vi "ResetMedia.vi"(8 "error in (no error)":errorcluster, 11 "UI Refs":T1) -> (0 "error out":errorcluster, 3 "UI Refs":T1)   [LabVIEW 2015]
uses:
  Controls & Type Defs/UI Data.ctl
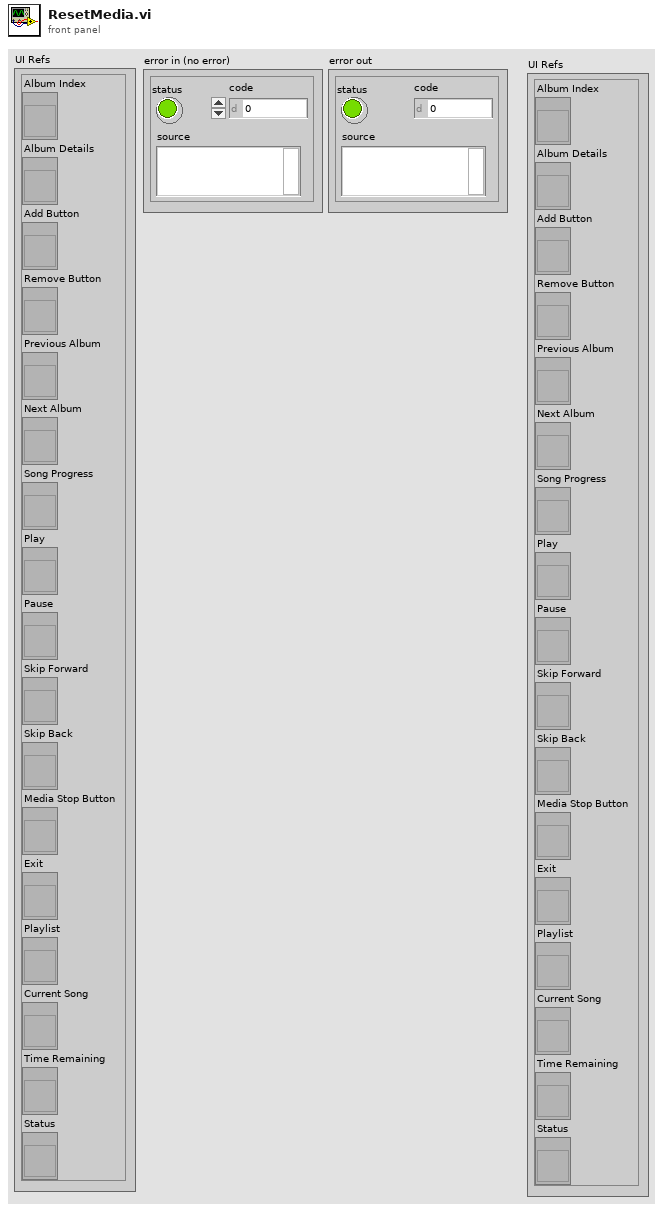
[diagram p1: front panel]
types:
  T1 = typedef "UI Data.ctl" = cluster{"Album Index":refnum<vi>, "Album Details":refnum<vi>, "Add Button":refnum<vi>, "Remove Button":refnum<vi>, "Previous Album":refnum<vi>, "Next Album":refnum<vi>, "Song Progress":refnum<vi>, "Play":refnum<vi>, "Pause ":refnum<vi>, "Skip Forward":refnum<vi>, "Skip Back":refnum<vi>, "Media Stop Button":refnum<vi>, "Exit":refnum<vi>, "Playlist":refnum<vi>, "Current Song":refnum<vi>, "Time Remaining":refnum<vi>, "Status":refnum<vi>}
  T2 = enum8{"Enabled", "Disabled", "Disabled and Grayed Out"}
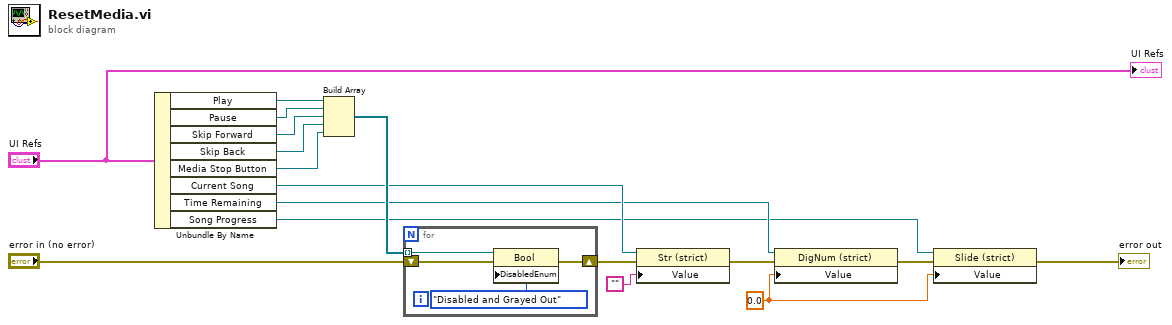
[diagram p0: block diagram]
diagram:
  w3 = 0.0 ("Value")
  n1 = Unbundle By Name("UI Refs") -> ("Play"=w17:refnum<vi>, "Pause"=w16:refnum<vi>, "Skip Forward"=w15:refnum<vi>, "Skip Back"=w14:refnum<vi>, "Media Stop Button"=w13:refnum<vi>, "Current Song"=w8:refnum<vi>, "Time Remaining"=w7:refnum<vi>, "Song Progress"=w4:refnum<vi>)
  n2 = Build Array(w17, w16, w15, w14, w13) -> (w12:refnum<vi>[])
  n3 = for {
    tunnel: w12 -> [w21] mode=indexing
    shift-right: [w19] -> w10
    shift-left: "error in (no error)" -> [w20]
    n4 = property class="Bool"(reference=w21, error in=w20, "DisabledEnum"=T2."Disabled and Grayed Out" ("Disabled")) -> (error out=w19:errorcluster)  [unwired: 1 out]
  }
  n5 = property class="Str (strict)"(reference=w8, error in=w10, "Value"="") -> (error out=w9:errorcluster)  [unwired: 1 out]
  n6 = property class="DigNum (strict)"(reference=w7, error in=w9, "Value"=w3) -> (error out=w5:errorcluster)  [unwired: 1 out]
  n7 = property class="Slide (strict)"(reference=w4, error in=w5, "Value"=w3) -> (error out=→"error out":errorcluster)  [unwired: 1 out]
  "UI Refs" <- "UI Refs"
